vi "USB2CNT_Test.vi"() -> ()   [LabVIEW 2010]
uses:
  sdk/api/Labview/USB2XXX.dll
panel:
  in  "停止":bool
  out "计数值":u32[](array[numeric])
  in  "PCNT_CONFIG":T1={"CounterMode"=0, "CounterPolarity"=1, "CounterBitWide"=16, "CounterPinMode"=1}
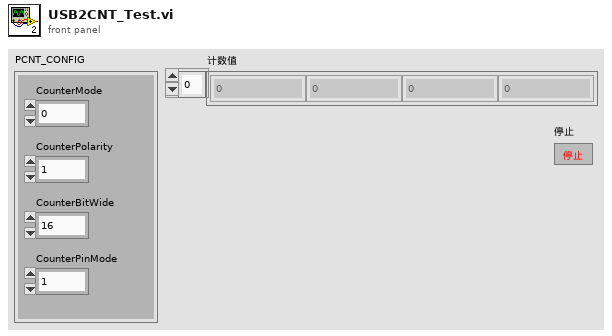
[diagram p1: front panel]
types:
  T1 = cluster{"CounterMode":u8, "CounterPolarity":i8, "CounterBitWide":u8, "CounterPinMode":u8}
  T2 = cluster{"CounterMode":u8, "CounterPolarity":i8, "CounterBitWide":u8, "CounterPinMode":u8}[]
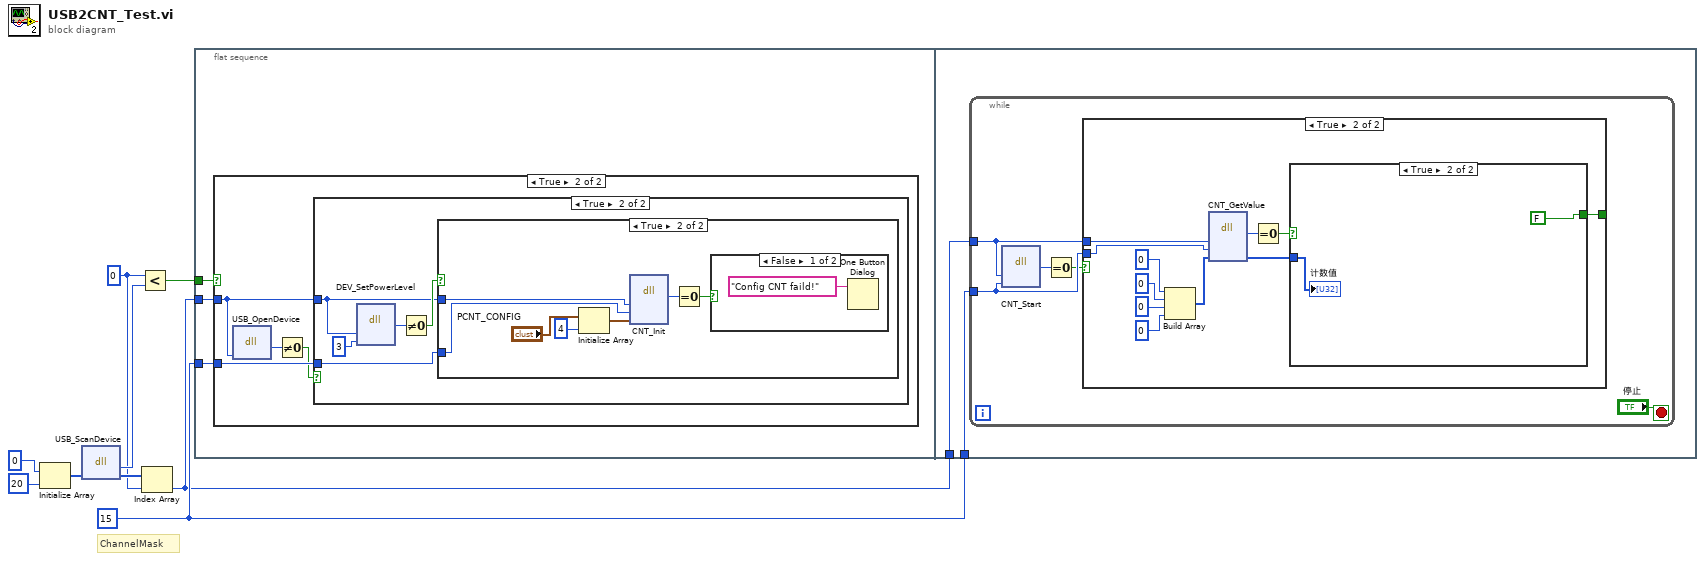
[diagram p0: block diagram]
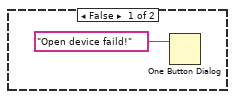
[diagram p4: hidden frame]
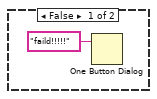
[diagram p6: hidden frame]
diagram:
  w2 = u8 15
  w4 = 0
  # "ChannelMask"
  n1 = Initialize Array(0, 20 ("dimension size")) -> (w9:i32[])
  n2 = dll-call lib="E:/OtherWork/STM32/USB2XXX_Example/sdk/api/Labview/USB2XXX.dll" fn="USB_ScanDevice"("pDevNum"=w9) -> ("return type"=w5:i32, "pDevNum"=w6:i32[])  [unwired: 3 in, 2 out]
  n3 = Less?(x=w4, y=w5) -> (x < y?=w3:bool)
  n4 = Index Array(array=w6, index=w4) -> (element=w1:i32)
  n5 = flat-sequence {
    tunnel: w3 -> [w12]
    tunnel: w1 -> [w11]
    tunnel: w2 -> [w10]
    tunnel: w2 -> [w31]
    tunnel: w1 -> [w32]
    frame #0 {
      n6 = case shown="True" w12 {
        tunnel: w11 -> [_ w14]
        tunnel: w10 -> [_ w16]
        frame False {
        }
        frame True {
          n7 = dll-call lib="E:/OtherWork/STM32/USB2XXX_Example/sdk/api/Labview/USB2XXX.dll" fn="USB_OpenDevice"("DevIndex"=w14) -> ("返回类型"=w13:u8)  [unwired: 4 in, 2 out]
          n8 = Not Equal To 0?(x=w13) -> (x != 0?=w15:bool)
          n9 = case shown="True" w15 {
            tunnel: w14 -> [_ w18]
            tunnel: w16 -> [_ w21]
            frame False {
            }
            frame True {
              n10 = dll-call lib="E:/OtherWork/STM32/USB2XXX_Example/sdk/api/Labview/USB2XXX.dll" fn="DEV_SetPowerLevel"("DevIndex"=w18, "PowerLevel"=u8 3 ("PuPd")) -> ("返回类型"=w17:u8)  [unwired: 5 in, 2 out]
              n11 = Not Equal To 0?(x=w17) -> (x != 0?=w20:bool)
              n12 = case shown="True" w20 {
                tunnel: w18 -> [_ w27]
                tunnel: w21 -> [_ w26]
                frame False {
                  n13 = One Button Dialog(message="Open device faild!") -> ()  [unwired: 1 in, 1 out]
                }
                frame True {
                  n14 = Initialize Array("PCNT_CONFIG", 4 ("dimension size")) -> (w24:T2)
                  n15 = dll-call lib="E:/OtherWork/STM32/USB2XXX_Example/sdk/api/Labview/USB2XXX.dll" fn="CNT_Init"("DevHandle"=w27, "ChannelMask"=w26, "PConfig"=w24) -> ("返回类型"=w29:i32)  [unwired: 6 in, 2 out]
                  n16 = Equal To 0?(x=w29) -> (x = 0?=w28:bool)
                  n17 = case shown="False" w28 {
                    frame False {
                      n18 = One Button Dialog(message="Config CNT faild!") -> ()  [unwired: 1 in, 1 out]
                    }
                    frame True {
                    }
                  }
                }
              }
            }
          }
        }
      }
    }
    frame #1 {
      n19 = while {
        tunnel: w32 -> [w37]
        tunnel: w31 -> [w36]
        stop <- "停止" stop-if-true
        n20 = dll-call lib="E:/OtherWork/STM32/USB2XXX_Example/sdk/api/Labview/USB2XXX.dll" fn="CNT_Start"("DevIndex"=w37, "ChannelMask"=w36) -> ("返回类型"=w35:u8)  [unwired: 5 in, 2 out]
        n21 = Equal To 0?(x=w35) -> (x = 0?=w34:bool)
        n22 = case shown="True" w34 {
          tunnel: w37 -> [_ w45]
          tunnel: w36 -> [_ w48]
          tunnel: [_ w42] -> _
          frame False {
            n23 = One Button Dialog(message="faild!!!!!") -> ()  [unwired: 1 in, 1 out]
          }
          frame True {
            n24 = Build Array(u32 0, u32 0 ("element"), u32 0 ("element"), u32 0 ("element")) -> (w44:u32[])
            n25 = dll-call lib="E:/OtherWork/STM32/USB2XXX_Example/sdk/api/Labview/USB2XXX.dll" fn="CNT_GetValue"("DevIndex"=w45, "ChannelMask"=w48, "pCntValues"=w44) -> ("返回类型"=w47:u8, "pCntValues"=w46:u32[])  [unwired: 5 in, 2 out]
            n26 = Equal To 0?(x=w47) -> (x = 0?=w43:bool)
            n27 = case shown="True" w43 {
              tunnel: w46 -> [_ w51]
              tunnel: [_ FALSE] -> w42
              frame False {
              }
              frame True {
                "计数值" <- w51
              }
            }
          }
        }
      }
    }
  }
